vi "error handler.vi"(7 "Status":enum16{"Init", "Read"}(ring)=enum."Read", 8 "error in (no error)":errorcluster, 10 "error":bool) -> (0 "error out":errorcluster, 2 "error":bool)   [LabVIEW 2014]
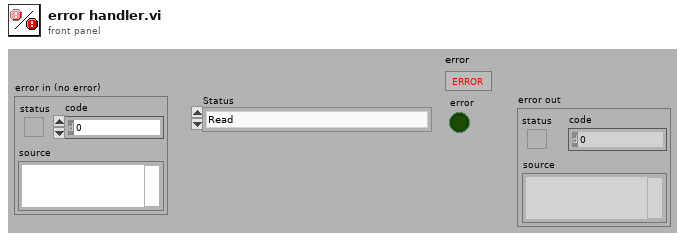
[diagram p1: front panel]
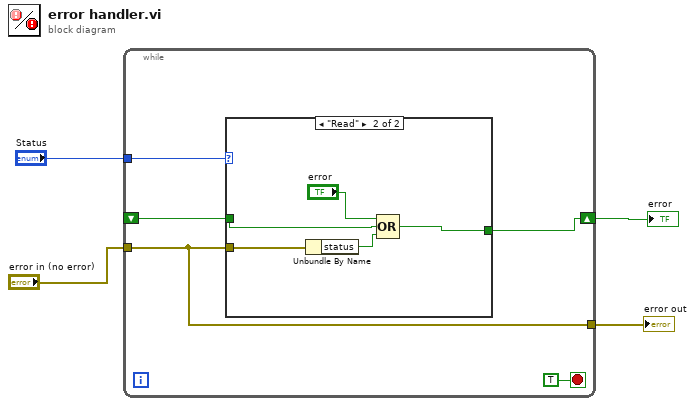
[diagram p0: block diagram]
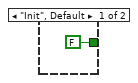
[diagram p2: hidden frame]
diagram:
  n1 = while {
    shift-right: [w7] -> w2
    shift-left: _ -> [w8]
    tunnel: "Status" -> [w9]
    tunnel: "error in (no error)" -> [w5]
    tunnel: [w5] -> w1
    stop <- TRUE stop-if-true
    n2 = case shown="\"Read\"" w9 {
      tunnel: w5 -> [_ w15]
      tunnel: w8 -> [_ w14]
      tunnel: [FALSE w12] -> w7
      frame "Init", Default {
      }
      frame "Read" {
        n3 = Unbundle By Name(w15) -> ("status"=w13:bool)
        n4 = Compound Arithmetic op=OR("error", w14, w13) -> (w12:bool)
      }
    }
  }
  "error" <- w2
  "error out" <- w1
